vi "Lab Panel V4.83.vi"() -> ()   [LabVIEW 2013]
uses:
  <vilib>/Platform/TimedLoop/XDataNode/timing_clust.ctl
  <vilib>/Platform/TimedLoop/XDataNode/nitl_modes.ctl
  <vilib>/Platform/TimedLoop/XDataNode/wakeup.ctl
  Global display 1.vi
  Global 1.vi
  Global display 3.vi
  Global display 2.vi
  <vilib>/platform/TimedLoop/XDataNode/XDataNode.xnode
  <vilib>/Platform/TimedLoop/XDataNode/XDNodeRunTimeDep.lvlib
panel:
  in  "stop all":bool
  in  "ADMIN":bool
  out "TEMP":bool
  out "AI":bool
  in  "Tab Control 2":T1(tab)
  out "SIG LAB05-2":T2 {"PF" format="%.2f"; "AMPS" format="%.1f"}
  out "SIG LAB05-1":T2 {"PF" format="%.2f"; "AMPS" format="%.1f"}
  out "SIG LAB04-2":T2 {"PF" format="%.2f"; "AMPS" format="%.1f"}
  out "SIG LAB04-1":T2 {"PF" format="%.2f"; "AMPS" format="%.1f"}
  out "SIG LAB03-2":T2 {"PF" format="%.2f"; "AMPS" format="%.1f"}
  out "SIG LAB03-1":T2 {"PF" format="%.2f"; "AMPS" format="%.1f"}
  out "SIG LAB02-2":T2 {"PF" format="%.2f"; "AMPS" format="%.1f"}
  in  "RUN LAB01-1":bool
  in  "O/I  LAB05-1":bool
  in  "O/I  LAB05-2":bool
  in  "O/I  LAB04-1":bool
  in  "O/I  LAB04-2":bool
  in  "O/I  LAB02-1":bool
  in  "O/I  LAB02-2":bool
  in  "O/I  LAB01-2":bool
  in  "O/I  LAB01-1":bool
  in  "O/I  LAB03-1":bool
  in  "RUN LAB05-2":bool
  in  "RUN LAB05-1":bool
  in  "RUN LAB04-2":bool
  in  "RUN LAB04-1":bool
  in  "RUN LAB03-2":bool
  in  "RUN LAB03-1":bool
  in  "RUN LAB02-2":bool
  in  "RUN LAB02-1":bool
  in  "RUN LAB01-2":bool
  in  "SELECT LAB05-2":T3(radio)
  in  "SELECT LAB05-1":T3(radio)
  in  "SELECT LAB04-2":T3(radio)
  in  "SELECT LAB04-1":T3(radio)
  in  "SELECT LAB03-2":T3(radio)
  in  "SELECT LAB03-1":T3(radio)
  in  "SELECT LAB02-2":T3(radio)
  in  "SELECT LAB02-1":T3(radio)
  in  "SELECT LAB01-2":T3(radio)
  in  "SELECT LAB01-1":T3(radio)
  in  "O/I  LAB03-2":bool
  out "SIG LAB01-1":T2 {"PF" format="%.2f"; "AMPS" format="%.1f"}
  out "SIG LAB01-2":T2 {"PF" format="%.2f"; "AMPS" format="%.1f"}
  out "SIG LAB02-1":T2 {"PF" format="%.2f"; "AMPS" format="%.1f"}
  out "DISP LAB05-2":T4 {"MINS" format="%.2g"}
  out "DISP LAB05-1":T4 {"MINS" format="%.2g"}
  out "DISP LAB04-2":T4 {"MINS" format="%.2g"}
  out "DISP LAB04-1":T4 {"MINS" format="%.2g"}
  out "DISP LAB03-2":T4 {"MINS" format="%.2g"}
  out "DISP LAB03-1":T4 {"MINS" format="%.2g"}
  in  "SET LAB05-2":T5={"NAME"="", "DESCRIPTION"="", "CYCLES"=5.0, "T-RISE mins"=0.0, "T-RISE deg C"=0.0} {"CYCLES" min=5.0 step=1.0}
  in  "SET LAB05-1":T5={"NAME"="", "DESCRIPTION"="", "CYCLES"=5.0, "T-RISE mins"=0.0, "T-RISE deg C"=0.0} {"CYCLES" min=5.0 step=1.0}
  in  "SET LAB04-2":T5={"NAME"="", "DESCRIPTION"="", "CYCLES"=5.0, "T-RISE mins"=0.0, "T-RISE deg C"=0.0} {"CYCLES" min=5.0 step=1.0}
  in  "SET LAB04-1":T5={"NAME"="", "DESCRIPTION"="", "CYCLES"=5.0, "T-RISE mins"=0.0, "T-RISE deg C"=0.0} {"CYCLES" min=5.0 step=1.0}
  in  "SET LAB03-2":T5={"NAME"="", "DESCRIPTION"="", "CYCLES"=5.0, "T-RISE mins"=0.0, "T-RISE deg C"=0.0} {"CYCLES" min=5.0 step=1.0}
  in  "SET LAB03-1":T5={"NAME"="", "DESCRIPTION"="", "CYCLES"=5.0, "T-RISE mins"=0.0, "T-RISE deg C"=0.0} {"CYCLES" min=5.0 step=1.0}
  out "DISP LAB02-2":T4 {"MINS" format="%.2g"}
  out "DISP LAB02-1":T4 {"MINS" format="%.2g"}
  in  "SET LAB02-2":T5={"NAME"="", "DESCRIPTION"="", "CYCLES"=5.0, "T-RISE mins"=0.0, "T-RISE deg C"=0.0} {"CYCLES" min=5.0 step=1.0}
  in  "SET LAB02-1":T5={"NAME"="", "DESCRIPTION"="", "CYCLES"=5.0, "T-RISE mins"=0.0, "T-RISE deg C"=0.0} {"CYCLES" min=5.0 step=1.0}
  out "RESULT LAB05-2":bool
  out "RESULT LAB05-1":bool
  out "RESULT LAB04-2":bool
  out "RESULT LAB04-1":bool
  out "RESULT LAB03-2":bool
  out "RESULT LAB03-1":bool
  out "RESULT LAB02-2":bool
  out "RESULT LAB02-1":bool
  out "RESULT LAB01-2":bool
  out "RESULT LAB01-1":bool
  in  "SET LAB01-1":T5={"NAME"="", "DESCRIPTION"="", "CYCLES"=5.0, "T-RISE mins"=0.0, "T-RISE deg C"=0.0} {"CYCLES" min=5.0 step=1.0}
  in  "SET LAB01-2":T5={"NAME"="", "DESCRIPTION"="", "CYCLES"=5.0, "T-RISE mins"=0.0, "T-RISE deg C"=0.0} {"CYCLES" min=5.0 step=1.0}
  out "DISP LAB01-1":T4 {"MINS" format="%.2g"}
  out "DISP LAB01-2":T4 {"MINS" format="%.2f"}
  out "TEMP RISE LAB05-2":cluster{"TL":dbl, "TN":dbl}
  out "TEMP RISE LAB05-1":cluster{"TL":dbl, "TN":dbl}
  out "TEMP RISE LAB04-2":cluster{"TL":dbl, "TN":dbl}
  out "TEMP RISE LAB04-1":cluster{"TL":dbl, "TN":dbl}
  out "TEMP RISE LAB03-2":cluster{"TL":dbl, "TN":dbl}
  out "TEMP RISE LAB03-1":cluster{"TL":dbl, "TN":dbl}
  out "TEMP RISE LAB02-2":cluster{"TL":dbl, "TN":dbl}
  out "TEMP RISE LAB02-1":cluster{"TL":dbl, "TN":dbl}
  out "TEMP RISE LAB01-2":cluster{"TL":dbl, "TN":dbl}
  out "TEMP RISE LAB01-1":cluster{"TL":dbl, "TN":dbl}
  in  "JIG OFF TIME (S)":dbl=2.0 min=2.0 max=10.0 step=0.5 format="%.1g"
  in  "JIG ON TIME (S)":dbl=1.0 min=1.0 max=10.0 step=0.5 format="%.1g"
  out "JIG LAB05-2":bool
  out "JIG LAB05-1":bool
  out "JIG LAB04-2":bool
  out "JIG LAB04-1":bool
  out "JIG LAB03-2":bool
  out "JIG LAB03-1":bool
  out "JIG LAB02-2":bool
  out "JIG LAB02-1":bool
  out "JIG LAB01-2":bool
  out "JIG LAB01-1":bool
  out "TEMP START LAB01-1":cluster{"TL":dbl, "TN":dbl}
  out "TEMP START LAB02-1":cluster{"TL":dbl, "TN":dbl}
  out "TEMP START LAB03-1":cluster{"TL":dbl, "TN":dbl}
  out "TEMP START LAB04-1":cluster{"TL":dbl, "TN":dbl}
  out "TEMP START LAB01-2":cluster{"TL":dbl, "TN":dbl}
  out "TEMP START LAB02-2":cluster{"TL":dbl, "TN":dbl}
  out "TEMP START LAB03-2":cluster{"TL":dbl, "TN":dbl}
  out "TEMP START LAB04-2":cluster{"TL":dbl, "TN":dbl}
  out "TEMP START LAB05-2":cluster{"TL":dbl, "TN":dbl}
  out "TEMP START LAB05-1":cluster{"TL":dbl, "TN":dbl}
  out "TEST VOLTS CHART":dynamicdata(graph)
  in  "Select  Cycle":enum32{"ON CYCLE", "OFF CYCLE"}(radio)
  out "TEST AMPS CHART":dynamicdata(graph)
  out "TEMPERATURE (L) CHART":dynamicdata(graph)
  out "TEMPERATURE (N) CHART":dynamicdata(graph)
  out "Message":string
  in  "MAIL SETTINGS":T6
  out "MAIL REPORT":string
  in  "TO (string):":string
  in  "Send Mail Now":bool
  in  "Auto Mail Send":bool
  in  "Network Directory":path
  out "JIG RELAY CYCLES":T7
  out "ON L05-2":cluster{"amps":dbl, "volts":dbl, "pf":dbl}
  out "ON L05-1":cluster{"amps":dbl, "volts":dbl, "pf":dbl}
  out "FAIL LAB05-2":cluster{"LO":dbl, "HI":dbl}
  out "FAIL LAB05-1":cluster{"LO":dbl, "HI":dbl}
  out "FAIL LAB04-2":cluster{"LO":dbl, "HI":dbl}
  out "FAIL LAB04-1":cluster{"LO":dbl, "HI":dbl}
  out "FAIL LAB03-2":cluster{"LO":dbl, "HI":dbl}
  out "FAIL LAB03-1":cluster{"LO":dbl, "HI":dbl}
  out "FAIL LAB02-2":cluster{"LO":dbl, "HI":dbl}
  out "FAIL LAB02-1":cluster{"LO":dbl, "HI":dbl}
  out "FAIL LAB01-2":cluster{"LO":dbl, "HI":dbl}
  out "FAIL LAB01-1":cluster{"LO":dbl, "HI":dbl}
  out "ON L01-1":cluster{"amps":dbl, "volts":dbl, "pf":dbl}
  out "ON L01-2":cluster{"amps":dbl, "volts":dbl, "pf":dbl}
  out "ON L02-1":cluster{"amps":dbl, "volts":dbl, "pf":dbl}
  out "ON L02-2":cluster{"amps":dbl, "volts":dbl, "pf":dbl}
  out "ON L03-1":cluster{"amps":dbl, "volts":dbl, "pf":dbl}
  out "ON L03-2":cluster{"amps":dbl, "volts":dbl, "pf":dbl}
  out "ON L04-1":cluster{"amps":dbl, "volts":dbl, "pf":dbl}
  out "ON L04-2":cluster{"amps":dbl, "volts":dbl, "pf":dbl}
  out "TEMP LA05":T8
  out "TEMP LA04":T8
  out "TEMP LA03":T8
  out "TEMP LA02":T8
  out "TEMP LA01":T8
  out "CAL LAB01":T9 {"2 (TN) cal" min=0.0 step=0.01 format="%.2f"; "2 (TL) cal" min=0.0 step=0.01 format="%.2f"; "2 (PF) cal" min=0.0 step=0.01 format="%.2f"; "2 (V) cal" min=0.0 step=0.01 format="%.2f"; "2 (A) cal" min=0.0 step=0.01 format="%.2f"; "1 (TN) cal" min=0.0 step=0.01 format="%.2f"; "1 (TL) cal" min=0.0 step=0.01 format="%.2f"; "1 (PF) cal" min=0.0 step=0.01 format="%.2f"; "1 (V) cal" min=0.0 step=0.01 format="%.2f"; "1  (A) cal" min=0.0 step=0.01 format="%.2f"}
  out "CAL LAB03":T9 {"2 (TN) cal" min=0.0 step=0.01 format="%.2f"; "2 (TL) cal" min=0.0 step=0.01 format="%.2f"; "2 (PF) cal" min=0.0 step=0.01 format="%.2f"; "2 (V) cal" min=0.0 step=0.01 format="%.2f"; "2 (A) cal" min=0.0 step=0.01 format="%.2f"; "1 (TN) cal" min=0.0 step=0.01 format="%.2f"; "1 (TL) cal" min=0.0 step=0.01 format="%.2f"; "1 (PF) cal" min=0.0 step=0.01 format="%.2f"; "1 (V) cal" min=0.0 step=0.01 format="%.2f"; "1  (A) cal" min=0.0 step=0.01 format="%.2f"}
  out "CAL LAB02":T10 {"2 (TN) cal" min=0.0 step=0.01 format="%.2f"; "2 (TL) cal" min=0.0 step=0.01 format="%.2f"; "2 (PF) cal" min=0.0 step=0.01 format="%.2f"; "2 (V) cal" min=0.0 step=0.01 format="%.2f"; "2 (A) cal" min=0.0 step=0.01 format="%.2f"; "1 (TN) cal" min=0.0 step=0.01 format="%.2f"; "1 (TL) cal" min=0.0 step=0.01 format="%.2f"; "1 (PF) cal" min=0.0 step=0.01 format="%.2f"; "1 (V) cal" min=0.0 step=0.01 format="%.2f"; "1 (A) cal" min=0.0 step=0.01 format="%.2f"}
  out "CAL LAB05":T9 {"2 (TN) cal" min=0.0 step=0.01 format="%.2f"; "2 (TL) cal" min=0.0 step=0.01 format="%.2f"; "2 (PF) cal" min=0.0 step=0.01 format="%.2f"; "2 (V) cal" min=0.0 step=0.01 format="%.2f"; "2 (A) cal" min=0.0 step=0.01 format="%.2f"; "1 (TN) cal" min=0.0 step=0.01 format="%.2f"; "1 (TL) cal" min=0.0 step=0.01 format="%.2f"; "1 (PF) cal" min=0.0 step=0.01 format="%.2f"; "1 (V) cal" min=0.0 step=0.01 format="%.2f"; "1  (A) cal" min=0.0 step=0.01 format="%.2f"}
  out "CAL LAB04":T9 {"2 (TN) cal" min=0.0 step=0.01 format="%.2f"; "2 (TL) cal" min=0.0 step=0.01 format="%.2f"; "2 (PF) cal" min=0.0 step=0.01 format="%.2f"; "2 (V) cal" min=0.0 step=0.01 format="%.2f"; "2 (A) cal" min=0.0 step=0.01 format="%.2f"; "1 (TN) cal" min=0.0 step=0.01 format="%.2f"; "1 (TL) cal" min=0.0 step=0.01 format="%.2f"; "1 (PF) cal" min=0.0 step=0.01 format="%.2f"; "1 (V) cal" min=0.0 step=0.01 format="%.2f"; "1  (A) cal" min=0.0 step=0.01 format="%.2f"}
  out "calibration file error out":errorcluster
  in  "CALIBRATE":bool
  in  "Temp Test Cal":dbl
  in  "Set Temp Lps":dbl
  out "Temp Loops":dbl
  in  "Fail Loops":dbl
  out "Save JC":bool
  out "simulate":bool
  in  "Temp Value":dbl
  in  "Temp Delay Lps":dbl
  in  "SAMPLES":dbl
  in  "RATE (Hz)":dbl
  in  "JIG TEST":T11
  in  "C drive data root dir":path
  out "run lab05-2":bool
  out "run lab05-1":bool
  out "run lab04-2":bool
  out "run lab04-1":bool
  out "run lab03-2":bool
  out "run lab03-1":bool
  out "run lab02-2":bool
  out "run lab02-1":bool
  out "run lab01-2":bool
  out "run lab01-1":bool
  in  "Tab Control":T12(tab)
  out "LAB01-2 (GRAPH)":dynamicdata(graph)
  out "LAB01-1 (GRAPH)":dynamicdata(graph)
  out "LAB02-2 (GRAPH)":dynamicdata(graph)
  out "LAB02-1 (GRAPH)":dynamicdata(graph)
  out "LAB03-2 (GRAPH)":dynamicdata(graph)
  out "LAB03-1 (GRAPH)":dynamicdata(graph)
  out "LAB04-2 (GRAPH)":dynamicdata(graph)
  out "LAB04-1 (GRAPH)":dynamicdata(graph)
  out "LAB05-2 (GRAPH)":dynamicdata(graph)
  out "LAB05-1 (GRAPH)":dynamicdata(graph)
  out "LAB05 TEMP":T13
  out "LAB04 TEMP":T13
  out "LAB02 TEMP":T13
  out "LAB01 TEMP":T13
  out "LAB03 TEMP":T13
  out "Analog Error Array":errorcluster[](array[cluster])
  out "AI loop time":dbl format="%.6g"
  out "loops":dbl
  in  "loop  delay(mS)":dbl
  out "on loops":dbl
  out "off loops":dbl
  out "jig cycle":dbl
  out "TDMS LAB01-1":refnum<k34>
  out "data file error":errorcluster
  out "TDMS LAB02-1":refnum<k34>
  out "TDMS LAB01-2":refnum<k34>
  out "TDMS LAB02-2":refnum<k34>
  out "TDMS LAB03-1":refnum<k34>
  out "TDMS LAB03-2":refnum<k34>
  out "TDMS LAB04-1":refnum<k34>
  out "TDMS LAB04-2":refnum<k34>
  out "TDMS LAB05-1":refnum<k34>
  out "TDMS LAB05-2":refnum<k34>
  out "mail control":string
  out "File Time Stamp":timestamp
  in  "stop":bool
  in  "Select COM port":refnum<visa-resource-name>="COM6"
  out "COM port":refnum<visa-resource-name>="COM6"
  # "LAB01"
  # "LAB02"
  # "LAB05"
  # "LAB03"
  # "LAB04"
  # "LAB01"
  # "LAB02"
  # "LAB03"
  # "LAB04"
  # "LAB05"
  # "JIG SET"
  # "(Enter recipients address seperated by comma)"
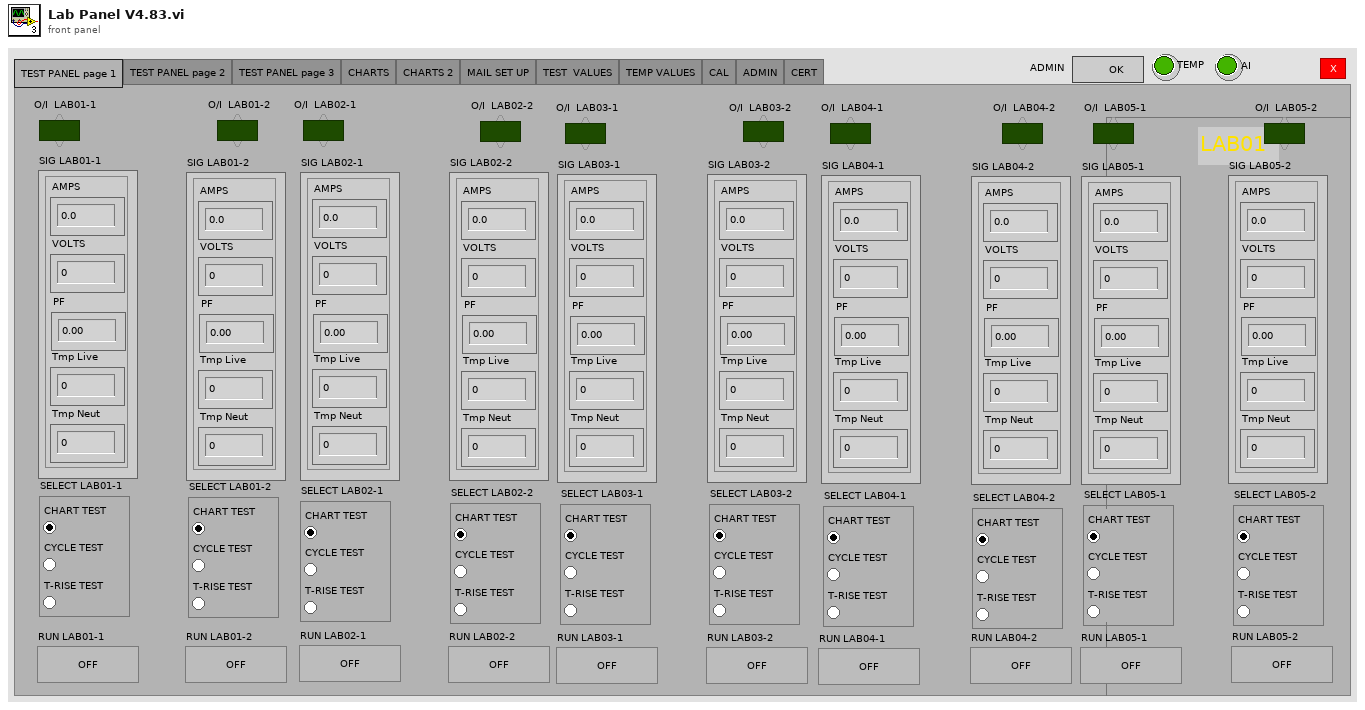
[diagram p1: front panel]
types:
  T1 = enum32{"TEST PANEL page 1", "TEST PANEL page 2", "TEST PANEL page 3", "CHARTS", "CHARTS 2", "MAIL SET UP", "TEST  VALUES", "TEMP VALUES", "CAL", "ADMIN", "CERT"}
  T2 = cluster{"AMPS":dbl, "VOLTS":dbl, "PF":dbl, "Tmp Live":dbl, "Tmp Neut":dbl}
  T3 = enum32{"CHART TEST", "CYCLE TEST", "T-RISE TEST"}
  T4 = cluster{"CYCLE":dbl, "MINS":dbl, "STATUS":string}
  T5 = cluster{"NAME":string, "DESCRIPTION":string, "CYCLES":dbl, "T-RISE mins":dbl, "T-RISE deg C":dbl}
  T6 = cluster{"OUT SERVER ADDRESS":string, "FROM ACCOUNT":string, "USER NAME":string, "PASSWORD":string, "TEST MAIL":bool, "TEST MAIL STATUS":string, "mail error":errorcluster}
  T7 = cluster{"LAB01-1":dbl, "LAB01-2":dbl, "LAB02-1":dbl, "LAB02-2":dbl, "LAB03-1":dbl, "LAB03-2":dbl, "LAB04-1":dbl, "LAB04-2":dbl, "LAB05-1":dbl, "LAB05-2":dbl}
  T8 = cluster{"TL-1":dbl, "TN-1":dbl, "TL-2":dbl, "TN-2":dbl, "TL -1COUNT":dbl, "TN-1 COUNT":dbl, "TL-2 COUNT":dbl, "TN-2 COUNT":dbl}
  T9 = cluster{"1  (A) cal":dbl, "1 (V) cal":dbl, "1 (PF) cal":dbl, "1 (TL) cal":dbl, "1 (TN) cal":dbl, "2 (A) cal":dbl, "2 (V) cal":dbl, "2 (PF) cal":dbl, "2 (TL) cal":dbl, "2 (TN) cal":dbl}
  T10 = cluster{"1 (A) cal":dbl, "1 (V) cal":dbl, "1 (PF) cal":dbl, "1 (TL) cal":dbl, "1 (TN) cal":dbl, "2 (A) cal":dbl, "2 (V) cal":dbl, "2 (PF) cal":dbl, "2 (TL) cal":dbl, "2 (TN) cal":dbl}
  T11 = cluster{" LAB01-1":bool, " LAB01-2":bool, "LAB02-1":bool, " LAB02-2":bool, "LAB03-1":bool, "LAB03-2":bool, "LAB04-1":bool, "LAB04-2":bool, "LAB05-1":bool, "LAB05-2":bool}
  T12 = enum32{"LAB01", "LAB02", "LAB03", "LAB04", "LAB05", "TEMPERATURE", "ERROR"}
  T13 = cluster{"T1 Live":dbl, "T1 Neut":dbl, "T2 Live":dbl, "T2 Neut":dbl, "ID":dbl, "ER":dbl}
  T14 = enum8{"Enabled", "Disabled", "Disabled and Grayed Out"}
  T15 = typedef "XDNodeRunTimeDep.lvlib/timing_clust.ctl" = cluster{"Expected End [f-1]":u64, "Actual End [f-1]":u64, "Finished Late? [f-1]":bool, "Expected End [i-1]":u64, "Actual End [i-1]":u64, "Finished Late? [i-1]":bool, "Expected Start [i]":u64, "Actual Start [i]":u64, "Expected Start [f]":u64, "Actual Start [f]":u64, "Source Name":string, "Structure Name":string, "Period":i64, "Deadline":i64, "Offset":i64, "Start":i64, "Priority":i32, "Timeout":i32, "Mode":T16, "Wakeup Reason":T17, "Error":errorcluster, "Source Type":string, "Secondary Source Type":string, "Global End Time":u64, "Global Start Time":u64, "Frame Duration":u64, "Iteration Duration":u64, "Assigned CPU":i32, "I/O Scan Engine Mode":u32}
  T16 = typedef "XDNodeRunTimeDep.lvlib/nitl_modes.ctl" = enum32{"No Change", "Process missed periods, maintain original phase", "Discard missed periods, maintain original phase", "Process missed periods, ignore original phase", "Discard missed periods, ignore original phase"}
  T17 = typedef "XDNodeRunTimeDep.lvlib/wakeup.ctl" = enum32{"Normal", "Aborted", "Asynchronous wakeup", "Timing source error", "Timed loop error", "Timeout"}
  T18 = enum16{"open", "open or create", "create or replace", "create", "open (read-only)"}
  T19 = enum16{"open", "replace", "create", "open or create", "replace or create", "replace or create with confirmation"}
  T20 = cluster{"SET LAB01-1":cluster{"NAME":string, "DESCRIPTION":string, "CYCLES":dbl, "T-RISE mins":dbl, "T-RISE deg C":dbl}, "SET LAB01-2":cluster{"NAME":string, "DESCRIPTION":string, "CYCLES":dbl, "T-RISE mins":dbl, "T-RISE deg C":dbl}, "SET LAB02-1":cluster{"NAME":string, "DESCRIPTION":string, "CYCLES":dbl, "T-RISE mins":dbl, "T-RISE deg C":dbl}, "SET LAB02-2":cluster{"NAME":string, "DESCRIPTION":string, "CYCLES":dbl, "T-RISE mins":dbl, "T-RISE deg C":dbl}, "SET LAB03-1":cluster{"NAME":string, "DESCRIPTION":string, "CYCLES":dbl, "T-RISE mins":dbl, "T-RISE deg C":dbl}, "SET LAB03-2":cluster{"NAME":string, "DESCRIPTION":string, "CYCLES":dbl, "T-RISE mins":dbl, "T-RISE deg C":dbl}, "SET LAB04-1":cluster{"NAME":string, "DESCRIPTION":string, "CYCLES":dbl, "T-RISE mins":dbl, "T-RISE deg C":dbl}, "SET LAB04-2":cluster{"NAME":string, "DESCRIPTION":string, "CYCLES":dbl, "T-RISE mins":dbl, "T-RISE deg C":dbl}, "SET LAB05-1":cluster{"NAME":string, "DESCRIPTION":string, "CYCLES":dbl, "T-RISE mins":dbl, "T-RISE deg C":dbl}, "SET LAB05-2":cluster{"NAME":string, "DESCRIPTION":string, "CYCLES":dbl, "T-RISE mins":dbl, "T-RISE deg C":dbl}, "Network Directory":path, "C drive data root dir":path, "RATE (Hz)":dbl, "SAMPLES":dbl, "Select COM port":refnum<visa-resource-name>, "Temp Delay Lps":dbl, "Temp Value":dbl, "Fail Loops":dbl, "Temp Test Cal":dbl, "Set Temp Lps":dbl}
  T21 = cluster{"MAIL SETTINGS":cluster{"OUT SERVER ADDRESS":string, "FROM ACCOUNT":string, "USER NAME":string, "PASSWORD":string, "TEST MAIL":bool, "TEST MAIL STATUS":string, "mail error":errorcluster}, "Auto Mail Send":bool, string}
  T22 = cluster{"T1":dbl, "T2":dbl, "T3":dbl, "T4":dbl, "ID":dbl, "ER":dbl}
  T23 = cluster{"LAB01-1 (A)":dbl, "LAB01-1 (V)":dbl, "LAB01-1 (PF)":dbl, "LAB01-2 (A)":dbl, "LAB01-2 (V)":dbl, "LAB01-2 (PF)":dbl}
  T24 = cluster{"LAB02-1 (A)":dbl, "LAB02-1 (V)":dbl, "LAB02-1 (PF)":dbl, "LAB02-2 (A)":dbl, "LAB02-2 (V)":dbl, "LAB02-2 (PF)":dbl}
  T25 = cluster{"LAB03-1 (A)":dbl, "LAB03-1 (V)":dbl, "LAB03-1 (PF)":dbl, "LAB03-2 (A)":dbl, "LAB03-2 (V)":dbl, "LAB03-2 (PF)":dbl}
  T26 = cluster{"LAB04-1 (A)":dbl, "LAB04-1 (V)":dbl, "LAB04-1 (PF)":dbl, "LAB04-2 (A)":dbl, "LAB04-2 (V)":dbl, "LAB04-2 (PF)":dbl}
  T27 = cluster{"LAB05-1 (A)":dbl, "LAB05-1 (V)":dbl, "LAB05-1 (PF)":dbl, "LAB05-2 (A)":dbl, "LAB05-2 (V)":dbl, "LAB05-2 (PF)":dbl}
  T28 = cluster{"FAIL LAB01-1":cluster{"LO":dbl, "HI":dbl}, "SIG LAB01-1":cluster{"AMPS":dbl, "VOLTS":dbl, "PF":dbl, "Tmp Live":dbl, "Tmp Neut":dbl}, "TEMP START LAB01-1":cluster{"TL":dbl, "TN":dbl}, "DISP LAB01-1":cluster{"CYCLE":dbl, "MINS":dbl, "STATUS":string}, "SET LAB01-1":cluster{"NAME":string, "DESCRIPTION":string, "CYCLES":dbl, "T-RISE mins":dbl, "T-RISE deg C":dbl}, "TDMS LAB01-1":refnum<k34>}
  T29 = cluster{"FAIL LAB01-2":cluster{"LO":dbl, "HI":dbl}, "SIG LAB01-2":cluster{"AMPS":dbl, "VOLTS":dbl, "PF":dbl, "Tmp Live":dbl, "Tmp Neut":dbl}, "TEMP START LAB01-2":cluster{"TL":dbl, "TN":dbl}, "DISP LAB01-2":cluster{"CYCLE":dbl, "MINS":dbl, "STATUS":string}, "SET LAB01-2":cluster{"NAME":string, "DESCRIPTION":string, "CYCLES":dbl, "T-RISE mins":dbl, "T-RISE deg C":dbl}, "TDMS LAB01-2":refnum<k34>}
  T30 = cluster{"FAIL LAB02-1":cluster{"LO":dbl, "HI":dbl}, "SIG LAB02-1":cluster{"AMPS":dbl, "VOLTS":dbl, "PF":dbl, "Tmp Live":dbl, "Tmp Neut":dbl}, "TEMP START LAB02-1":cluster{"TL":dbl, "TN":dbl}, "DISP LAB02-1":cluster{"CYCLE":dbl, "MINS":dbl, "STATUS":string}, "SET LAB02-1":cluster{"NAME":string, "DESCRIPTION":string, "CYCLES":dbl, "T-RISE mins":dbl, "T-RISE deg C":dbl}, "TDMS LAB02-1":refnum<k34>}
  T31 = cluster{"FAIL LAB02-2":cluster{"LO":dbl, "HI":dbl}, "SIG LAB02-2":cluster{"AMPS":dbl, "VOLTS":dbl, "PF":dbl, "Tmp Live":dbl, "Tmp Neut":dbl}, "TEMP START LAB02-2":cluster{"TL":dbl, "TN":dbl}, "DISP LAB02-2":cluster{"CYCLE":dbl, "MINS":dbl, "STATUS":string}, "SET LAB02-2":cluster{"NAME":string, "DESCRIPTION":string, "CYCLES":dbl, "T-RISE mins":dbl, "T-RISE deg C":dbl}, "TDMS LAB02-2":refnum<k34>}
  T32 = cluster{"FAIL LAB03-1":cluster{"LO":dbl, "HI":dbl}, "SIG LAB03-1":cluster{"AMPS":dbl, "VOLTS":dbl, "PF":dbl, "Tmp Live":dbl, "Tmp Neut":dbl}, "TEMP START LAB03-1":cluster{"TL":dbl, "TN":dbl}, "DISP LAB03-1":cluster{"CYCLE":dbl, "MINS":dbl, "STATUS":string}, "SET LAB03-1":cluster{"NAME":string, "DESCRIPTION":string, "CYCLES":dbl, "T-RISE mins":dbl, "T-RISE deg C":dbl}, "TDMS LAB03-1":refnum<k34>}
  T33 = cluster{"FAIL LAB03-2":cluster{"LO":dbl, "HI":dbl}, "SIG LAB03-2":cluster{"AMPS":dbl, "VOLTS":dbl, "PF":dbl, "Tmp Live":dbl, "Tmp Neut":dbl}, "TEMP START LAB03-2":cluster{"TL":dbl, "TN":dbl}, "DISP LAB03-2":cluster{"CYCLE":dbl, "MINS":dbl, "STATUS":string}, "SET LAB03-2":cluster{"NAME":string, "DESCRIPTION":string, "CYCLES":dbl, "T-RISE mins":dbl, "T-RISE deg C":dbl}, "TDMS LAB03-2":refnum<k34>}
  T34 = cluster{"FAIL LAB04-1":cluster{"LO":dbl, "HI":dbl}, "SIG LAB04-1":cluster{"AMPS":dbl, "VOLTS":dbl, "PF":dbl, "Tmp Live":dbl, "Tmp Neut":dbl}, "TEMP START LAB04-1":cluster{"TL":dbl, "TN":dbl}, "DISP LAB04-1":cluster{"CYCLE":dbl, "MINS":dbl, "STATUS":string}, "SET LAB04-1":cluster{"NAME":string, "DESCRIPTION":string, "CYCLES":dbl, "T-RISE mins":dbl, "T-RISE deg C":dbl}, "TDMS LAB04-1":refnum<k34>}
  T35 = cluster{"FAIL LAB04-2":cluster{"LO":dbl, "HI":dbl}, "SIG LAB04-2":cluster{"AMPS":dbl, "VOLTS":dbl, "PF":dbl, "Tmp Live":dbl, "Tmp Neut":dbl}, "TEMP START LAB04-2":cluster{"TL":dbl, "TN":dbl}, "DISP LAB04-2":cluster{"CYCLE":dbl, "MINS":dbl, "STATUS":string}, "SET LAB04-2":cluster{"NAME":string, "DESCRIPTION":string, "CYCLES":dbl, "T-RISE mins":dbl, "T-RISE deg C":dbl}, "TDMS LAB04-2":refnum<k34>}
  T36 = cluster{"FAIL LAB05-1":cluster{"LO":dbl, "HI":dbl}, "SIG LAB05-1":cluster{"AMPS":dbl, "VOLTS":dbl, "PF":dbl, "Tmp Live":dbl, "Tmp Neut":dbl}, "TEMP START LAB05-1":cluster{"TL":dbl, "TN":dbl}, "DISP LAB05-1":cluster{"CYCLE":dbl, "MINS":dbl, "STATUS":string}, "SET LAB05-1":cluster{"NAME":string, "DESCRIPTION":string, "CYCLES":dbl, "T-RISE mins":dbl, "T-RISE deg C":dbl}, "TDMS LAB05-1":refnum<k34>}
  T37 = cluster{"FAIL LAB05-2":cluster{"LO":dbl, "HI":dbl}, "SIG LAB05-2":cluster{"AMPS":dbl, "VOLTS":dbl, "PF":dbl, "Tmp Live":dbl, "Tmp Neut":dbl}, "TEMP START LAB05-2":cluster{"TL":dbl, "TN":dbl}, "DISP LAB05-2":cluster{"CYCLE":dbl, "MINS":dbl, "STATUS":string}, "SET LAB05-2":cluster{"NAME":string, "DESCRIPTION":string, "CYCLES":dbl, "T-RISE mins":dbl, "T-RISE deg C":dbl}, "TDMS LAB05-2":refnum<k34>}
  T38 = cluster{"MAIL SETTINGS":cluster{"OUT SERVER ADDRESS":string, "FROM ACCOUNT":string, "USER NAME":string, "PASSWORD":string, "TEST MAIL":bool, "TEST MAIL STATUS":string, "mail error":errorcluster}, "Auto Mail Send":bool, "TO (string):":string}
  T39 = cluster{"TP1-L":dbl, "TP1-N":dbl, "TP2-L":dbl, "TP2-N":dbl, "TP1-L COUNT":dbl, "TP1-N COUNT":dbl, "TP2-L COUNT":dbl, "TP2-N COUNT":dbl}
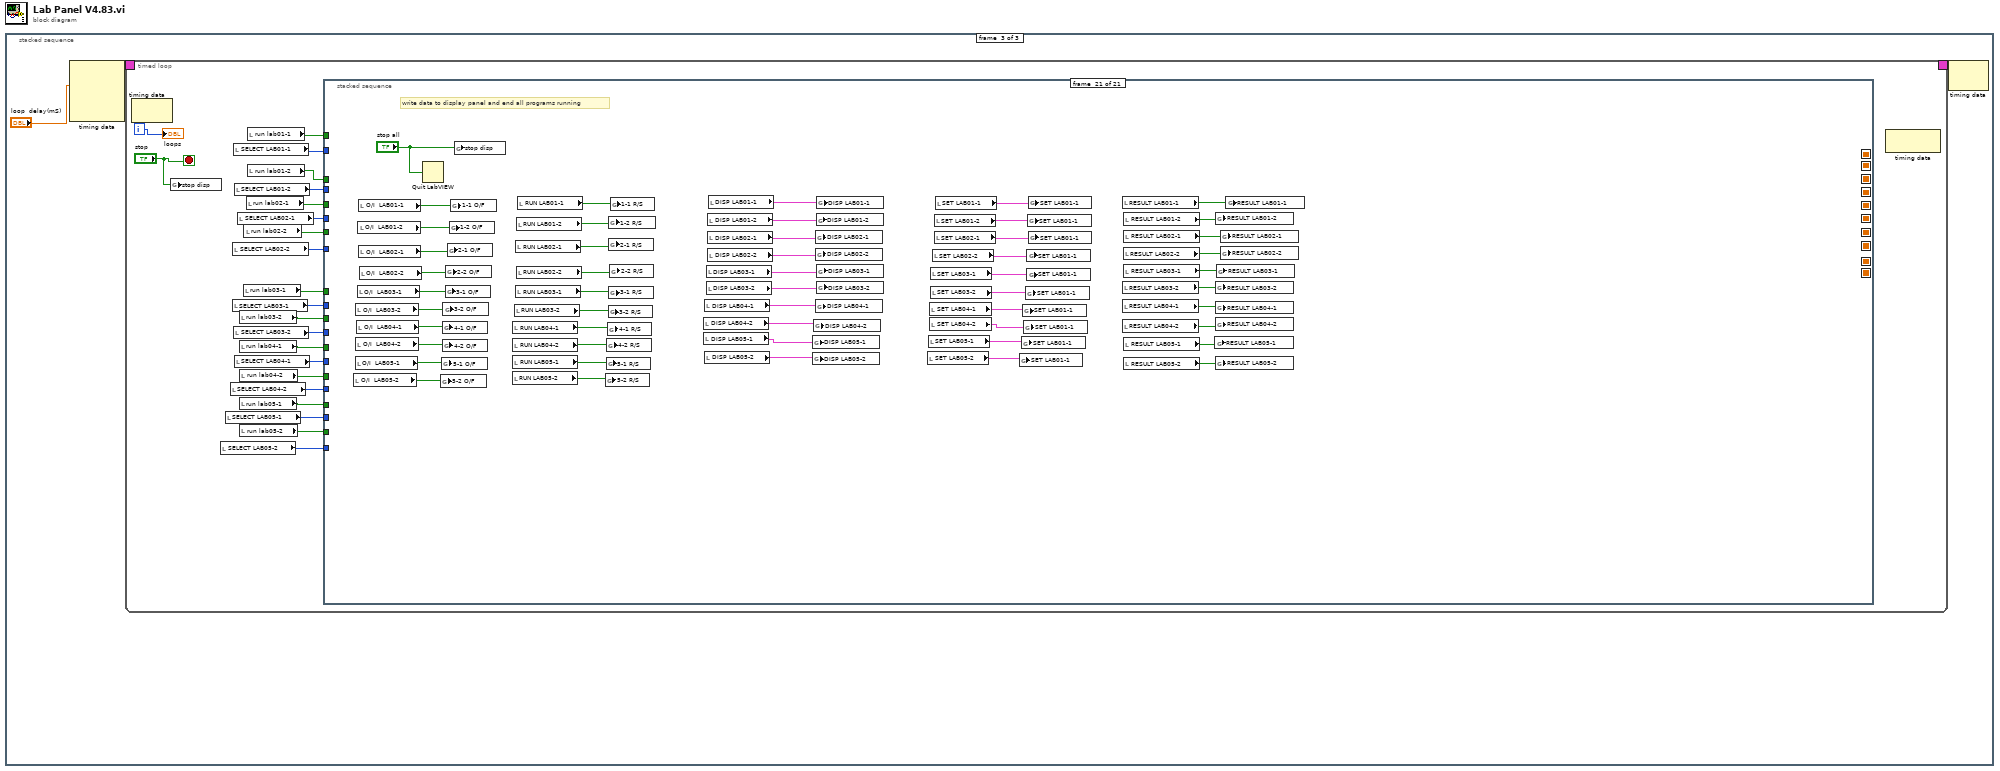
[diagram p0: block diagram]
diagram:
  n1 = stacked-sequence {
    frame #0 {
      n2 = local write "loop  delay(mS)"(500) -> ()
      n3 = local write "Save JC"(FALSE) -> ()
      "jig cycle" <- 0
    }
    frame #1 {
      # "do 1st time set up"
      n4 = stacked-sequence {
        frame #0 {
          # "disable front panel while 1st time set up is being done"
          n5 = disable-structure shown="Disabled" {
            frame Disabled {
              n6 = property on="Tab Control 2" class="TabCtl (strict)"() -> ("Pages"=w10:refnum<vi>[])  [unwired: 2 in, 2 out]
              n7 = Index Array(array=w10, index=9) -> (element=w8:refnum<vi>)
              n8 = property class="Page"(reference=w8, "PageVis"=FALSE) -> ()  [unwired: 1 in, 2 out]
            }
            frame Enabled {
            }
          }
          n9 = property on="Tab Control 2" class="TabCtl (strict)"("Value"=0) -> ()  [unwired: 2 in, 2 out]
          n10 = local write "ADMIN"(FALSE) -> ()
          n11 = property on="Tab Control 2" class="TabCtl (strict)"("DisabledEnum"=T14."Disabled and Grayed Out" ("Disabled")) -> ()  [unwired: 2 in, 2 out]
        }
        frame #1 {
          # "get calibration values"
          n12 = call "sub vi - get calibration values v1.vi"() -> ("LAB01 (CAL)"=→"CAL LAB01":T9, "LAB02 (CAL)"=→"CAL LAB02":T10, "LAB03 (CAL)"=→"CAL LAB03":T9, "LAB04 (CAL)"=→"CAL LAB04":T9, "calibration file error out"=→"calibration file error out":errorcluster, "LAB05 (CAL)"=→"CAL LAB05":T9)  [unwired: 10 in]
        }
        frame #2 {
          # "get last saved test settings from file"
          n13 = local read "Network Directory"() -> (w35:path)
          n14 = local read "C drive data root dir"() -> (w33:path)
          n15 = local read "SET LAB05-2"() -> (w65:T5)
          n16 = local read "SET LAB05-1"() -> (w66:T5)
          n17 = local read "SAMPLES"() -> (w31:dbl)
          n18 = local read "SET LAB04-2"() -> (w67:T5)
          n19 = local read "RATE (Hz)"() -> (w32:dbl)
          n20 = local read "SET LAB03-2"() -> (w64:T5)
          n21 = local read "SET LAB04-1"() -> (w68:T5)
          n22 = local read "SET LAB03-1"() -> (w63:T5)
          n23 = local read "SET LAB02-2"() -> (w62:T5)
          n24 = local read "SET LAB02-1"() -> (w61:T5)
          n25 = local read "SET LAB01-2"() -> (w60:T5)
          n26 = local read "SET LAB01-1"() -> (w59:T5)
          n27 = local read "Select COM port"() -> (w27:refnum<visa-resource-name>)
          n28 = local read "Temp Delay Lps"() -> (w26:dbl)
          n29 = local read "Temp Value"() -> (w25:dbl)
          n30 = local read "Temp Test Cal"() -> (w20:dbl)
          n31 = local read "Set Temp Lps"() -> (w19:dbl)
          n32 = local read "Fail Loops"() -> (w22:dbl)
          n33 = Bundle("SET LAB01-1"=w59, "SET LAB01-2"=w60, "SET LAB02-1"=w61, "SET LAB02-2"=w62, "SET LAB03-1"=w63, "SET LAB03-2"=w64, "SET LAB04-1"=w68, "SET LAB04-2"=w67, "SET LAB05-1"=w66, "SET LAB05-2"=w65, "Network Directory"=w35, "C drive data root dir"=w33, "RATE (Hz)"=w32, "SAMPLES"=w31, "Select COM port"=w27, "Temp Delay Lps"=w26, "Temp Value"=w25, "Fail Loops"=w22, "Temp Test Cal"=w20, "Set Temp Lps"=w19) -> (w52:T20)  [unwired: 1 in]
          n34 = String To Path(string="c:\\crabtree\\Set Up\\") -> (path=w56:path)
          n35 = Build Path(base path=w56, name or relative path="settings.bin") -> (appended path=w54:path)
          n36 = Create Folder(path (use dialog)=w56) -> (error out=w58:errorcluster)  [unwired: 2 in, 2 out]
          n37 = call <vilib>:"Clear Errors.vi"("error in (no error)"=w58) -> ()  [unwired: 6 in, 1 out]
          n38 = Open/Create/Replace File(file path (use dialog)=w54) -> (refnum out=w51:refnum<file>, error out=w53:errorcluster)  [unwired: 5 in, 1 out]
          n39 = Read from Binary File(5:w52, 8:w53, 11:w51) -> (0:w48:errorcluster, 2:w50:T20, 3:w49:refnum<file>)  [unwired: 3 in, 1 out]
          n40 = Unbundle(w50) -> ("SET LAB01-1"=w46:T5, "SET LAB01-2"=w45:T5, "SET LAB02-1"=w44:T5, "SET LAB02-2"=w43:T5, "SET LAB03-1"=w42:T5, "SET LAB03-2"=w41:T5, "SET LAB04-1"=w40:T5, "SET LAB04-2"=w39:T5, "SET LAB05-1"=w38:T5, "SET LAB05-2"=w37:T5, "Network Directory"=w36:path, "C drive data root dir"=w34:path, "RATE (Hz)"=w29:dbl, "SAMPLES"=w30:dbl, "Select COM port"=w28:refnum<visa-resource-name>, "Temp Delay Lps"=w24:dbl, "Temp Value"=w23:dbl, "Fail Loops"=w21:dbl, "Temp Test Cal"=w18:dbl, "Set Temp Lps"=w17:dbl)
          n41 = Close File(refnum=w49, error in=w48) -> (error out=w47:errorcluster)  [unwired: 1 out]
          n42 = local write "data file error"(w47) -> ()
          n43 = local write "Temp Test Cal"(w18) -> ()
          n44 = local write "Set Temp Lps"(w17) -> ()
          n45 = local write "Fail Loops"(w21) -> ()
          n46 = local write "Temp Delay Lps"(w24) -> ()
          n47 = local write "C drive data root dir"(w34) -> ()
          n48 = local write "Temp Value"(w23) -> ()
          n49 = local write "Select COM port"(w28) -> ()
          n50 = local write "Network Directory"(w36) -> ()
          n51 = local write "SAMPLES"(w30) -> ()
          n52 = local write "RATE (Hz)"(w29) -> ()
          n53 = local write "SET LAB04-2"(w39) -> ()
          n54 = local write "SET LAB05-1"(w38) -> ()
          n55 = local write "SET LAB04-1"(w40) -> ()
          n56 = local write "SET LAB05-2"(w37) -> ()
          n57 = local write "SET LAB02-1"(w44) -> ()
          n58 = local write "SET LAB02-2"(w43) -> ()
          n59 = local write "SET LAB03-1"(w42) -> ()
          n60 = local write "SET LAB03-2"(w41) -> ()
          n61 = local write "SET LAB01-1"(w46) -> ()
          n62 = local write "SET LAB01-2"(w45) -> ()
        }
        frame #3 {
          # "get last saved jig cycles value from file"
          n63 = String To Path(string="c:\\crabtree\\Jig Cycles\\") -> (path=w78:path)
          n64 = Build Path(base path=w78, name or relative path="jigcycles.bin") -> (appended path=w76:path)
          n65 = Create Folder(path (use dialog)=w78) -> (error out=w80:errorcluster)  [unwired: 2 in, 2 out]
          n66 = call <vilib>:"Clear Errors.vi"("error in (no error)"=w80) -> ()  [unwired: 6 in, 1 out]
          n67 = Open/Create/Replace File(file path (use dialog)=w76) -> (refnum out=w74:refnum<file>, error out=w75:errorcluster)  [unwired: 5 in, 1 out]
          n68 = Read from Binary File(5:T7 {"LAB01-1"=0.0, "LAB01-2"=0.0, "LAB02-1"=0.0, "LAB02-2"=0.0, "LAB03-1"=0.0, "LAB03-2"=0.0, "LAB04-1"=0.0, "LAB04-2"=0.0, "LAB05-1"=0.0, "LAB05-2"=0.0} ("JIG RELAY CYCLES"), 8:w75, 11:w74) -> (0:w72:errorcluster, 2:w69:T7, 3:w73:refnum<file>)  [unwired: 3 in, 1 out]
          n69 = local write "JIG RELAY CYCLES"(w69) -> ()
          n70 = Close File(refnum=w73, error in=w72) -> (error out=w71:errorcluster)  [unwired: 1 out]
          n71 = local write "data file error"(w71) -> ()
        }
        frame #4 {
          # "get mail settings"
          n72 = local read "Auto Mail Send"() -> (w84:bool)
          n73 = local read "MAIL SETTINGS"() -> (w88:T6)
          n74 = String To Path(string="c:\\crabtree\\Set Up\\") -> (path=w96:path)
          n75 = Build Path(base path=w96, name or relative path="mail.bin") -> (appended path=w94:path)
          n76 = Create Folder(path (use dialog)=w96) -> (error out=w98:errorcluster)  [unwired: 2 in, 2 out]
          n77 = Bundle("MAIL SETTINGS"=w88, "Auto Mail Send"=w84, "") -> (w87:T21)  [unwired: 1 in]
          n78 = call <vilib>:"Clear Errors.vi"("error in (no error)"=w98) -> ()  [unwired: 6 in, 1 out]
          n79 = Open/Create/Replace File(file path (use dialog)=w94) -> (refnum out=w92:refnum<file>, error out=w93:errorcluster)  [unwired: 5 in, 1 out]
          n80 = Read from Binary File(5:w87, 8:w93, 11:w92) -> (0:w90:errorcluster, 2:w86:T21, 3:w91:refnum<file>)  [unwired: 3 in, 1 out]
          n81 = Unbundle(w86) -> ("MAIL SETTINGS"=w85:T6, "Auto Mail Send"=w83:bool, w82:string)
          n82 = local write "TO (string):"(w82) -> ()
          n83 = local write "Auto Mail Send"(w83) -> ()
          n84 = local write "MAIL SETTINGS"(w85) -> ()
          n85 = Close File(refnum=w91, error in=w90) -> (error out=w89:errorcluster)  [unwired: 1 out]
          n86 = local write "data file error"(w89) -> ()
        }
        frame #5 {
          # "set display status if blank"
          n87 = local read "DISP LAB03-2"() -> (w128:T4)
          n88 = local read "DISP LAB03-1"() -> (w135:T4)
          n89 = local read "DISP LAB02-2"() -> (w142:T4)
          n90 = local read "DISP LAB01-2"() -> (w155:T4)
          n91 = local read "DISP LAB01-1"() -> (w164:T4)
          n92 = local read "DISP LAB02-1"() -> (w149:T4)
          n93 = Unbundle(w128) -> ("STATUS"=w130:string)  [unwired: 2 out]
          n94 = Unbundle(w135) -> ("STATUS"=w137:string)  [unwired: 2 out]
          n95 = Unbundle(w142) -> ("STATUS"=w144:string)  [unwired: 2 out]
          n96 = Unbundle(w149) -> ("STATUS"=w151:string)  [unwired: 2 out]
          n97 = Unbundle(w155) -> ("STATUS"=w158:string)  [unwired: 2 out]
          n98 = Unbundle(w164) -> ("STATUS"=w165:string)  [unwired: 2 out]
          n99 = Equal?(x="", y=w130) -> (x = y?=w132:bool)
          n100 = Equal?(x="", y=w137) -> (x = y?=w139:bool)
          n101 = Equal?(x="", y=w144) -> (x = y?=w146:bool)
          n102 = Equal?(x="", y=w151) -> (x = y?=w153:bool)
          n103 = Equal?(x="", y=w158) -> (x = y?=w160:bool)
          n104 = Equal?(x="", y=w165) -> (x = y?=w167:bool)
          n105 = Select(t="STOP", s=w132, f=w130) -> (s? t:f=w129:string)
          n106 = Select(t="STOP", s=w139, f=w137) -> (s? t:f=w136:string)
          n107 = Select(t="STOP", s=w146, f=w144) -> (s? t:f=w143:string)
          n108 = Select(t="STOP", s=w153, f=w151) -> (s? t:f=w150:string)
          n109 = Select(t="STOP", s=w160, f=w158) -> (s? t:f=w157:string)
          n110 = Select(t="STOP", s=w167, f=w165) -> (s? t:f=w163:string)
          n111 = Bundle(cluster=w128, "STATUS"=w129) -> (w127:T4)  [unwired: 2 in]
          n112 = Bundle(cluster=w135, "STATUS"=w136) -> (w134:T4)  [unwired: 2 in]
          n113 = Bundle(cluster=w142, "STATUS"=w143) -> (w141:T4)  [unwired: 2 in]
          n114 = Bundle(cluster=w149, "STATUS"=w150) -> (w148:T4)  [unwired: 2 in]
          n115 = Bundle(cluster=w155, "STATUS"=w157) -> (w156:T4)  [unwired: 2 in]
          n116 = Bundle(cluster=w164, "STATUS"=w163) -> (w162:T4)  [unwired: 2 in]
          n117 = local write "DISP LAB01-2"(w156) -> ()
          n118 = local write "DISP LAB01-1"(w162) -> ()
          n119 = local write "DISP LAB02-1"(w148) -> ()
          n120 = local write "DISP LAB03-1"(w134) -> ()
          n121 = local write "DISP LAB02-2"(w141) -> ()
          n122 = local write "DISP LAB03-2"(w127) -> ()
          n123 = local read "DISP LAB05-2"() -> (w100:T4)
          n124 = local read "DISP LAB05-1"() -> (w107:T4)
          n125 = local read "DISP LAB04-2"() -> (w109:T4)
          n126 = local read "DISP LAB04-1"() -> (w111:T4)
          n127 = Unbundle(w100) -> ("STATUS"=w102:string)  [unwired: 2 out]
          n128 = Unbundle(w107) -> ("STATUS"=w113:string)  [unwired: 2 out]
          n129 = Unbundle(w109) -> ("STATUS"=w118:string)  [unwired: 2 out]
          n130 = Unbundle(w111) -> ("STATUS"=w123:string)  [unwired: 2 out]
          n131 = Equal?(x="", y=w102) -> (x = y?=w104:bool)
          n132 = Equal?(x="", y=w113) -> (x = y?=w115:bool)
          n133 = Equal?(x="", y=w118) -> (x = y?=w120:bool)
          n134 = Equal?(x="", y=w123) -> (x = y?=w125:bool)
          n135 = Select(t="STOP", s=w104, f=w102) -> (s? t:f=w101:string)
          n136 = Select(t="STOP", s=w115, f=w113) -> (s? t:f=w112:string)
          n137 = Select(t="STOP", s=w120, f=w118) -> (s? t:f=w117:string)
          n138 = Select(t="STOP", s=w125, f=w123) -> (s? t:f=w122:string)
          n139 = Bundle(cluster=w100, "STATUS"=w101) -> (w99:T4)  [unwired: 2 in]
          n140 = Bundle(cluster=w107, "STATUS"=w112) -> (w106:T4)  [unwired: 2 in]
          n141 = Bundle(cluster=w109, "STATUS"=w117) -> (w108:T4)  [unwired: 2 in]
          n142 = Bundle(cluster=w111, "STATUS"=w122) -> (w110:T4)  [unwired: 2 in]
          n143 = local write "DISP LAB05-2"(w99) -> ()
          n144 = local write "DISP LAB05-1"(w106) -> ()
          n145 = local write "DISP LAB04-1"(w110) -> ()
          n146 = local write "DISP LAB04-2"(w108) -> ()
        }
        frame #6 {
          # "initialise analog input express vi's"
          n147 = for {
            N: 2.0 -> [_]
            n148 = call "sub vi - analog 1st setup v1.vi"() -> ("error out"=w171:errorcluster)  [unwired: 11 in, 4 out]
            n149 = Unbundle(w171) -> ("status"=w170:bool)  [unwired: 2 out]
            n150 = local write "simulate"(w170) -> ()
          }
        }
        frame #7 {
          # "get initial temperature values"
          n151 = stacked-sequence {
            frame #0 {
              w210 = TRUE
              n152 = local read "simulate"() -> (w172:bool)
              n153 = call "sub vi - GET ALL TEMP v5.vi"("LA01-EN"=w210, "simulate"=w172, "LA02-EN"=w210, "LA03-EN"=w210, "LA04-EN"=w210, "LA05-EN"=w210, "Gen Cal Value"=1) -> ("LA01 TEMP"=w208:T22, "LA02 TEMP"=w201:T22, "LA03 TEMP"=w194:T22, "LA04 TEMP"=w187:T22, "LA05 TEMP"=w180:T22)  [unwired: 3 in, 1 out]
              n154 = local write "LAB05 TEMP"(w180) -> ()
              n155 = local write "LAB04 TEMP"(w187) -> ()
              n156 = local write "LAB01 TEMP"(w208) -> ()
              n157 = local write "LAB02 TEMP"(w201) -> ()
              n158 = local write "LAB03 TEMP"(w194) -> ()
              n159 = Unbundle(w194) -> ("T1"=w191:dbl, "T2"=w190:dbl, "T3"=w189:dbl, "T4"=w188:dbl)  [unwired: 2 out]
              n160 = Unbundle(w208) -> ("T1"=w206:dbl, "T2"=w205:dbl, "T3"=w204:dbl, "T4"=w203:dbl)  [unwired: 2 out]
              n161 = Unbundle(w201) -> ("T1"=w198:dbl, "T2"=w197:dbl, "T3"=w196:dbl, "T4"=w195:dbl)  [unwired: 2 out]
              n162 = Unbundle(w187) -> ("T1"=w185:dbl, "T2"=w184:dbl, "T3"=w183:dbl, "T4"=w182:dbl)  [unwired: 2 out]
              n163 = Unbundle(w180) -> ("T1"=w178:dbl, "T2"=w177:dbl, "T3"=w176:dbl, "T4"=w175:dbl)  [unwired: 2 out]
              n164 = local read "TEMP LA05"() -> (w179:T8)
              n165 = local read "TEMP LA04"() -> (w186:T8)
              n166 = local write "Temp Loops"(0) -> ()
              n167 = local read "TEMP LA02"() -> (w200:T8)
              n168 = local read "TEMP LA03"() -> (w193:T8)
              n169 = local read "TEMP LA01"() -> (w207:T8)
              n170 = Bundle(cluster=w193, "TL-1"=w191, "TN-1"=w190, "TL-2"=w189, "TN-2"=w188) -> (w192:T8)  [unwired: 4 in]
              n171 = Bundle(cluster=w207, "TL-1"=w206, "TN-1"=w205, "TL-2"=w204, "TN-2"=w203) -> (w202:T8)  [unwired: 4 in]
              n172 = Bundle(cluster=w200, "TL-1"=w198, "TN-1"=w197, "TL-2"=w196, "TN-2"=w195) -> (w199:T8)  [unwired: 4 in]
              n173 = Bundle(cluster=w186, "TL-1"=w185, "TN-1"=w184, "TL-2"=w183, "TN-2"=w182) -> (w181:T8)  [unwired: 4 in]
              n174 = Bundle(cluster=w179, "TL-1"=w178, "TN-1"=w177, "TL-2"=w176, "TN-2"=w175) -> (w174:T8)  [unwired: 4 in]
              n175 = local write "TEMP LA03"(w192) -> ()
              n176 = local write "TEMP LA01"(w202) -> ()
              n177 = local write "TEMP LA02"(w199) -> ()
              n178 = local write "TEMP LA05"(w174) -> ()
              n179 = local write "TEMP LA04"(w181) -> ()
            }
            frame #1 {
              w211 = 0
              n180 = local read "LAB01 TEMP"() -> (w217:T13)
              n181 = Unbundle By Name(w217) -> ("T1 Live"=w216:dbl, "T1 Neut"=w215:dbl, "T2 Live"=w214:dbl, "T2 Neut"=w213:dbl)  [unwired: 2 out]
              n182 = local read "TEMP LA01"() -> (w218:T8)
              n183 = Bundle By Name(cluster=w218, "TL-1"=w216, "TN-1"=w215, "TL-2"=w214, "TN-2"=w213, "TL -1COUNT"=w211, "TN-1 COUNT"=w211, "TL-2 COUNT"=w211, "TN-2 COUNT"=w211) -> (w212:T8)
              n184 = local write "TEMP LA01"(w212) -> ()
            }
            frame #2 {
              w219 = 0
              n185 = local read "LAB02 TEMP"() -> (w225:T13)
              n186 = Unbundle By Name(w225) -> ("T1 Live"=w224:dbl, "T1 Neut"=w223:dbl, "T2 Live"=w222:dbl, "T2 Neut"=w221:dbl)  [unwired: 2 out]
              n187 = local read "TEMP LA02"() -> (w226:T8)
              n188 = Bundle By Name(cluster=w226, "TL-1"=w224, "TN-1"=w223, "TL-2"=w222, "TN-2"=w221, "TL -1COUNT"=w219, "TN-1 COUNT"=w219, "TL-2 COUNT"=w219, "TN-2 COUNT"=w219) -> (w220:T8)
              n189 = local write "TEMP LA02"(w220) -> ()
            }
            frame #3 {
              w227 = 0
              n190 = local read "LAB03 TEMP"() -> (w233:T13)
              n191 = Unbundle By Name(w233) -> ("T1 Live"=w232:dbl, "T1 Neut"=w231:dbl, "T2 Live"=w230:dbl, "T2 Neut"=w229:dbl)  [unwired: 2 out]
              n192 = local read "TEMP LA03"() -> (w234:T8)
              n193 = Bundle By Name(cluster=w234, "TL-1"=w232, "TN-1"=w231, "TL-2"=w230, "TN-2"=w229, "TL -1COUNT"=w227, "TN-1 COUNT"=w227, "TL-2 COUNT"=w227, "TN-2 COUNT"=w227) -> (w228:T8)
              n194 = local write "TEMP LA03"(w228) -> ()
            }
            frame #4 {
              w235 = 0
              n195 = local read "LAB04 TEMP"() -> (w241:T13)
              n196 = Unbundle By Name(w241) -> ("T1 Live"=w240:dbl, "T1 Neut"=w239:dbl, "T2 Live"=w238:dbl, "T2 Neut"=w237:dbl)  [unwired: 2 out]
              n197 = local read "TEMP LA04"() -> (w242:T8)
              n198 = Bundle By Name(cluster=w242, "TL-1"=w240, "TN-1"=w239, "TL-2"=w238, "TN-2"=w237, "TL -1COUNT"=w235, "TN-1 COUNT"=w235, "TL-2 COUNT"=w235, "TN-2 COUNT"=w235) -> (w236:T8)
              n199 = local write "TEMP LA04"(w236) -> ()
            }
            frame #5 {
              w243 = 0
              n200 = local read "LAB05 TEMP"() -> (w249:T13)
              n201 = Unbundle By Name(w249) -> ("T1 Live"=w248:dbl, "T1 Neut"=w247:dbl, "T2 Live"=w246:dbl, "T2 Neut"=w245:dbl)  [unwired: 2 out]
              n202 = local read "TEMP LA05"() -> (w250:T8)
              n203 = Bundle By Name(cluster=w250, "TL-1"=w248, "TN-1"=w247, "TL-2"=w246, "TN-2"=w245, "TL -1COUNT"=w243, "TN-1 COUNT"=w243, "TL-2 COUNT"=w243, "TN-2 COUNT"=w243) -> (w244:T8)
              n204 = local write "TEMP LA05"(w244) -> ()
            }
          }
        }
        frame #8 {
          # "enable front panel, all settings done"
          n205 = property on="Tab Control 2" class="TabCtl (strict)"("DisabledEnum"=T14."Enabled" ("Disabled")) -> ()  [unwired: 2 in, 2 out]
          n206 = property on="Tab Control 2" class="TabCtl (strict)"("Value"=0) -> ()  [unwired: 2 in, 2 out]
        }
        frame #9 {
          # "check network directory valid"
          n207 = while {
            stop <- w255 continue-if-true
            w253 = TRUE
            n208 = local read "Network Directory"() -> (w257:path)
            n209 = property on="Tab Control 2" class="TabCtl (strict)"("Value"=5) -> ()  [unwired: 2 in, 2 out]
            n210 = File/Directory Info(path=w257) -> (error out=w258:errorcluster)  [unwired: 1 in, 6 out]
            n211 = Unbundle(w258) -> ("status"=w255:bool)  [unwired: 2 out]
            n212 = case shown="True" w255 {
              frame False {
                n213 = local write "Message"("") -> ()
              }
              frame True {
                "Message" <- "NETWORK DIRECTORY NOT FOUND!!!!"
              }
            }
            n214 = property on="Message" class="Str"("Text.TextColor"=u32 16711680) -> ()  [unwired: 2 in, 2 out]
